vi "LS_BRIGT.vi"(8 "error in (no error)":errorcluster, 9 "Brightness":enum16{"25%", "50%", "75%", "100%"}(ring), 10 "Data Cluster In":T3 {"GUI Data Cluster"."SBR" format="%08b"}, 11 "Config Cluster In":T1={"General"={"Config.ini"=path "", "Default Logging Path"=path ""}, "Hardware"={"Measure Rate (1/s)"=0, "HP DMM VISA"="", "LS 335 VISA"="", "HP DM"={"Range"=enum."Autorange", "Autozero"=FALSE, "Display"=enum."3 1/2 Digit", "Blank LCD"=FALSE}, "LS335"={"Brightness"=enum."25%"}}, "Operation"={"Operation Mode"=enum."Logging", "Status"="", "NewLog?"=FALSE, "OvenWarn"=FALSE, "LS335"={"Heater A"=enum."Off", "Heater B"=enum."Off"}}}) -> (0 "error out":errorcluster, 2 "Data Cluster Out":T3 {"GUI Data Cluster"."SBR" format="%08b"}, 3 "Config Cluster Out":T1={"General"={"Config.ini"=path "", "Default Logging Path"=path ""}, "Hardware"={"Measure Rate (1/s)"=0, "HP DMM VISA"="", "LS 335 VISA"="", "HP DM"={"Range"=enum."Autorange", "Autozero"=FALSE, "Display"=enum."3 1/2 Digit", "Blank LCD"=FALSE}, "LS335"={"Brightness"=enum."25%"}}, "Operation"={"Operation Mode"=enum."Idle-Off", "Status"="", "NewLog?"=FALSE, "OvenWarn"=FALSE, "LS335"={"Heater A"=enum."Off", "Heater B"=enum."Off"}}}, 5 "return count":u32)   [LabVIEW 2021]
uses:
  Config_Cluster.ctl
  Mode_Enum.ctl
  Data_Cluster.ctl
  Measurement_Cluster.ctl
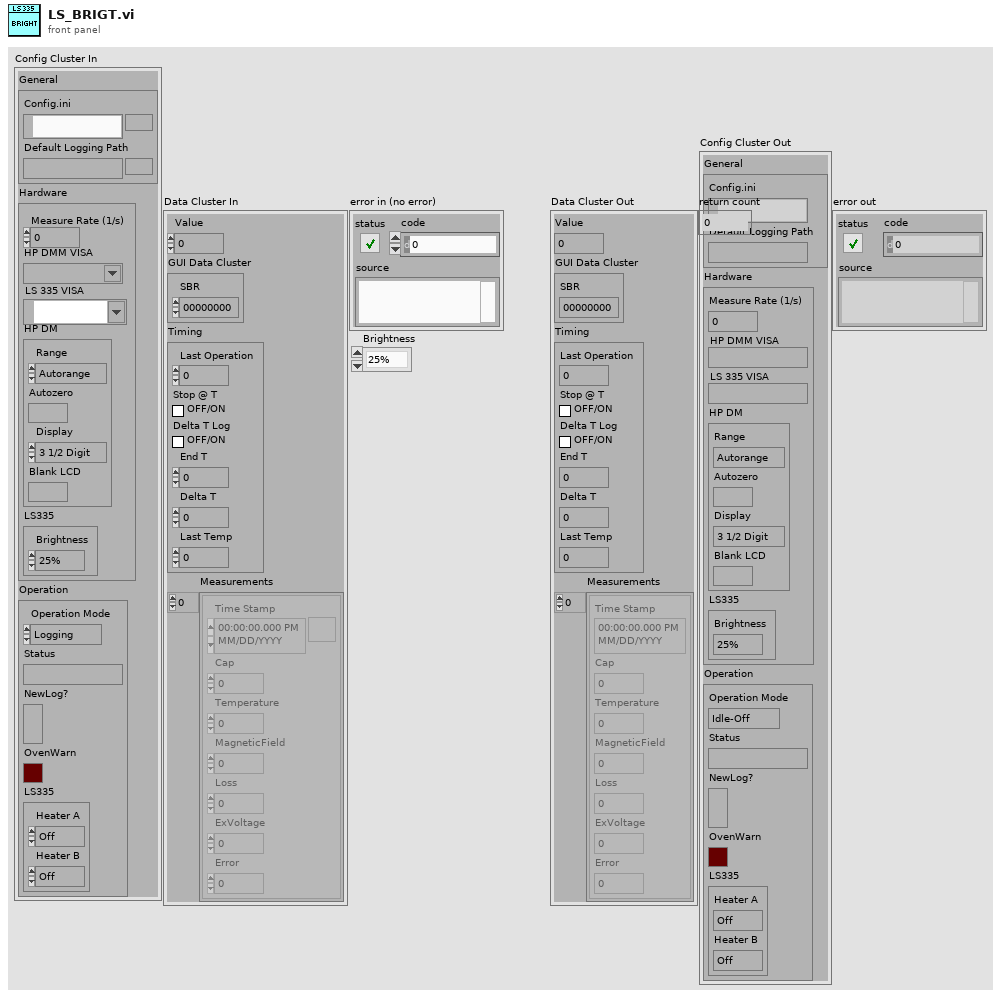
[diagram p1: front panel]
types:
  T1 = typedef "Config_Cluster.ctl" = cluster{"General":cluster{"Config.ini":path, "Default Logging Path":path}, "Hardware":cluster{"Measure Rate (1/s)":i32, "HP DMM VISA":refnum<visa-resource-name>, "LS 335 VISA":refnum<visa-resource-name>, "HP DM":cluster{"Range":enum16{"Autorange", "30mV", "300mV", "3V", "30V"}, "Autozero":bool, "Display":enum16{"3 1/2 Digit", "4 1/2 Digit", "5 1/2 Digit"}, "Blank LCD":bool}, "LS335":cluster{"Brightness":enum16{"25%", "50%", "75%", "100%"}}}, "Operation":cluster{"Operation Mode":T2, "Status":string, "NewLog?":bool, "OvenWarn":bool, "LS335":cluster{"Heater A":enum16{"Off", "Low", "Medium", "High"}, "Heater B":enum16{"Off", "Low", "Medium", "High"}}}}
  T2 = typedef "Mode_Enum.ctl" = enum16{"OvenNRDY", "Logging", "Idle-Off", "Idle"}
  T3 = typedef "Data_Cluster.ctl" = cluster{"Value":dbl, "GUI Data Cluster":cluster{"SBR":u16}, "Timing":cluster{"Last Operation":dbl, "Stop @ T":bool, "Delta T Log":bool, "End T":dbl, "Delta T":dbl, "Last Temp":dbl}, "Measurements":T4[]}
  T4 = typedef "Measurement_Cluster.ctl" = cluster{"Time Stamp":timestamp, "Cap":dbl, "Temperature":dbl, "MagneticField":dbl, "Loss":dbl, "ExVoltage":dbl, "Error":dbl}
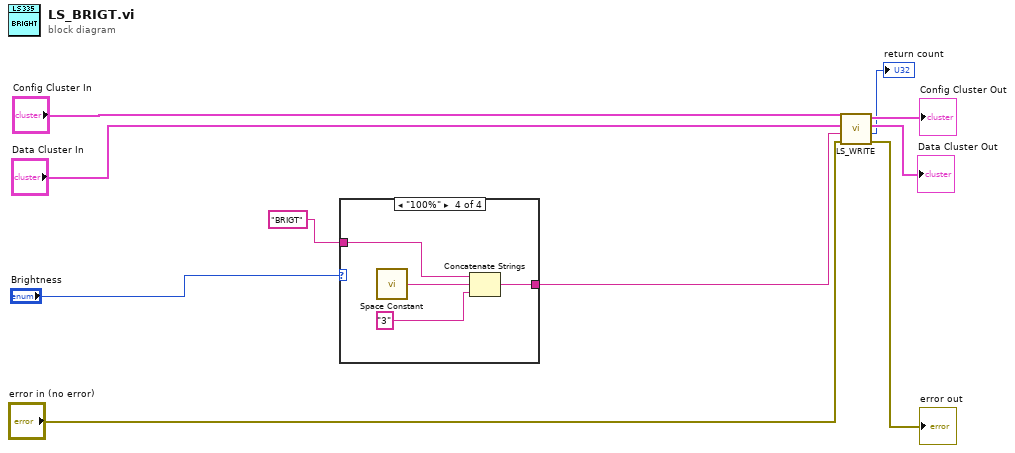
[diagram p0: block diagram]
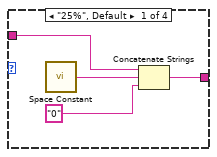
[diagram p2: hidden frame]
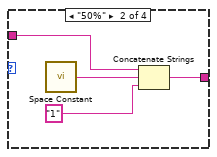
[diagram p3: hidden frame]
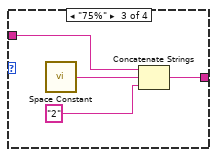
[diagram p4: hidden frame]
diagram:
  n1 = case shown="\"100%\"" "Brightness" {
    tunnel: "BRIGT" -> [w14 w18 w22 w26]
    tunnel: [w11 w15 w19 w23] -> w1
    frame "25%", Default {
      n2 = call <vilib>:"Space Constant.vi"() -> ("String"=w13:string)
      n3 = Concatenate Strings(w14, w13, "0") -> (w11:string)
    }
    frame "50%" {
      n4 = call <vilib>:"Space Constant.vi"() -> ("String"=w17:string)
      n5 = Concatenate Strings(w18, w17, "1") -> (w15:string)
    }
    frame "75%" {
      n6 = call <vilib>:"Space Constant.vi"() -> ("String"=w21:string)
      n7 = Concatenate Strings(w22, w21, "2") -> (w19:string)
    }
    frame "100%" {
      n8 = call <vilib>:"Space Constant.vi"() -> ("String"=w25:string)
      n9 = Concatenate Strings(w26, w25, "3") -> (w23:string)
    }
  }
  n10 = call "LS_WRITE.vi"("error in (no error)"="error in (no error)", "write buffer"=w1, "Data Cluster In"="Data Cluster In", "Config Cluster In"="Config Cluster In") -> ("error out"=→"error out":errorcluster, "return count"=→"return count":u32, "Data Cluster Out"=→"Data Cluster Out":T3, "Config Cluster Out"=→"Config Cluster Out":T1)  [unwired: 4 in]
